vi "save_config_file.vi"(8 "error in (no error)":errorcluster, 9 "config cluster variant":variant, 11 "GenericPlugin in":refnum<class "DataCollectionMG091001IntrinsicImaging.lvclass">) -> (0 "error out":errorcluster, 3 "GenericPlugin out":refnum<class "DataCollectionMG091001IntrinsicImaging.lvclass">)   [LabVIEW 2010]
uses:
  DataCollectionMG091001IntrinsicImaging.lvclass
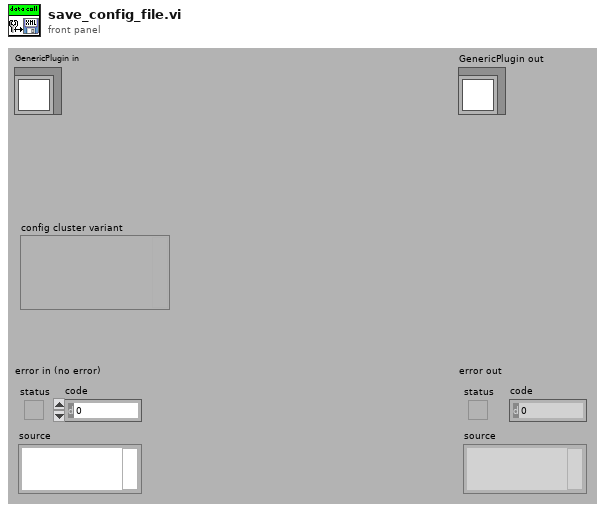
[diagram p1: front panel]
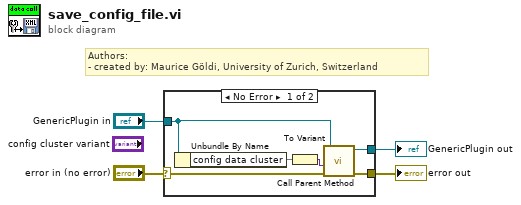
[diagram p0: block diagram]
diagram:
  # "Authors: \n- created by: Maurice Göldi, University of Zurich, Switzerland"
  n1 = case shown="No Error" "error in (no error)" {
    selector: "error in (no error)" -> [w8 w12]
    tunnel: [w10 w12] -> w4
    tunnel: [w9 w11] -> w3
    tunnel: "GenericPlugin in" -> [w7 w11]
    frame No Error {
      n2 = Unbundle By Name(w7) -> ("config data cluster"=w5)
      n3 = To Variant(anything=w5) -> (Variant=w6:variant)
      n4 = call-parent "Call Parent Method"("error in (no error)"=w8, 9:w6, "GenericPlugin in"=w7) -> ("error out"=w10:errorcluster, "GenericPlugin out"=w9:refnum<class "DataCollectionMG091001IntrinsicImaging.lvclass">)  [unwired: 7 in]
    }
    frame Error {
    }
  }
  "error out" <- w4
  "GenericPlugin out" <- w3
